vi "Get Number 9.vi"(9 "Number 6":string, 10 "Digit 5":string, 11 "Array":string[][](array[string])) -> (3 "Number 9":string)   [LabVIEW 2019, in "Day 8.lvlib"]
uses:
  Day 8.lvlib
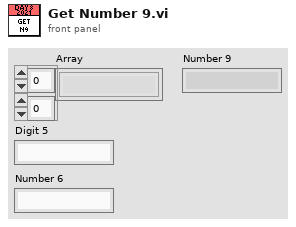
[diagram p1: front panel]
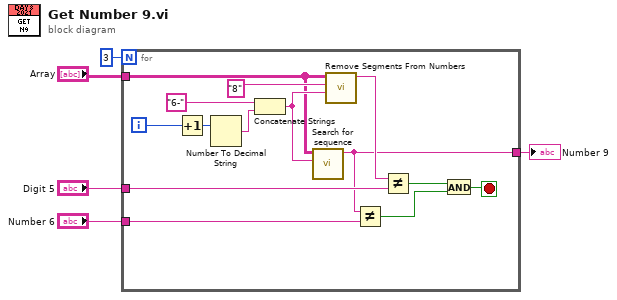
[diagram p0: block diagram]
diagram:
  n1 = for {
    N: 3 -> [_]
    tunnel: "Array" -> [w9]
    tunnel: "Digit 5" -> [w14]
    tunnel: "Number 6" -> [w8]
    tunnel: [w6] -> w1
    i -> [w16]
    stop <- w11 stop-if-true
    n2 = Increment(x=w16) -> (x+1=w17:i32)
    n3 = Number To Decimal String(number=w17) -> (decimal integer string=w18:string)  [unwired: 1 in]
    n4 = Concatenate Strings("6-" ("Pattern For Number Of Letters A"), w18) -> (w10:string)
    n5 = call "Search for sequence.vi"("Pattern For Number Of Letters"=w10, "Array"=w9) -> ("sequence"=w6:string)  [unwired: 9 in]
    n6 = call "Remove Segments From Numbers.vi"("Pattern For Letter Of Letters B"=w10, "Pattern For Number Of Letters A"="8", "Array"=w9) -> ("Result"=w13:string)  [unwired: 8 in]
    n7 = Not Equal?(x=w6, y=w8) -> (x != y?=w7:bool)
    n8 = Not Equal?(x=w13, y=w14) -> (x != y?=w12:bool)
    n9 = And(x=w12, y=w7) -> (x .and. y?=w11:bool)
  }
  "Number 9" <- w1
